vi "Gray Code to Binary.vi"(1 "Gray Code":i32[](array[numeric])) -> (0 "Binary Out":i32[](array[numeric]))   [LabVIEW 2018]
doc: "Converts a 1D array of gray-code data to binary"
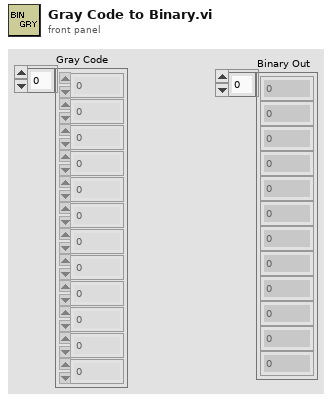
[diagram p1: front panel]
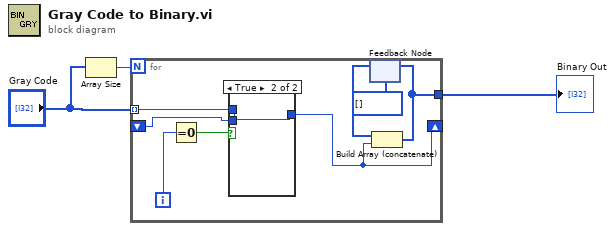
[diagram p0: block diagram]
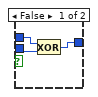
[diagram p2: hidden frame]
diagram:
  n1 = Array Size(array="Gray Code") -> (size(s)=w3:i32)
  n2 = for {
    N: w3 -> [_]
    tunnel: "Gray Code" -> [w10] mode=indexing
    shift-right: [w5] -> _
    shift-left: _ -> [w9]
    tunnel: [w7] -> w1
    i -> [w8]
    n3 = Equal To 0?(x=w8) -> (x = 0?=w11:bool)
    n4 = case shown="True" w11 {
      tunnel: [w13 w15] -> w5
      tunnel: w10 -> [w14 w15]
      tunnel: w9 -> [w12 _]
      frame False {
        n5 = Exclusive Or(1:w12, 2:w14) -> (0:w13:i32)
      }
      frame True {
      }
    }
    n6 = feedback #1(i32[] []) -> (w6:i32[])
    n7 = Build Array (concatenate)(w6, w5) -> (w7:i32[])
    n8 = feedback-in #1(w7) -> ()
  }
  "Binary Out" <- w1
